vi "_attribute_read_double.vi"(5 "Repeated Capability":string, 7 "Attribute":T1={"Identifier"="", "Descriptive Name"="", "Data Type"=enum."Integer 32", "Command"="", "Access"=enum."Read/Write", "Range Table"="", "Read Callback"="", "Write Callback"="", "Supported Models"="", "Instrument Options"="", "Index"=0, "OPC Wait"=FALSE, "No Status Check"=FALSE, "Cache Only"=FALSE}, 8 "error in":errorcluster caption="error in (no error)", 10 "Query Parameter":string, 11 "VISA resource name":refnum<visa-resource-name>) -> (0 "error out":errorcluster, 2 "Double out":dbl, 3 "VISA resource name out":refnum<visa-resource-name>)   [LabVIEW 2022 SP3, in "hmp4000_rsidr_core.lvlib"]
uses:
  hmp4000_rsidr_core.lvlib
  type_Attribute.ctl
  type_Attribute_Data_Type.ctl
  type_ReadWriteAccess.ctl
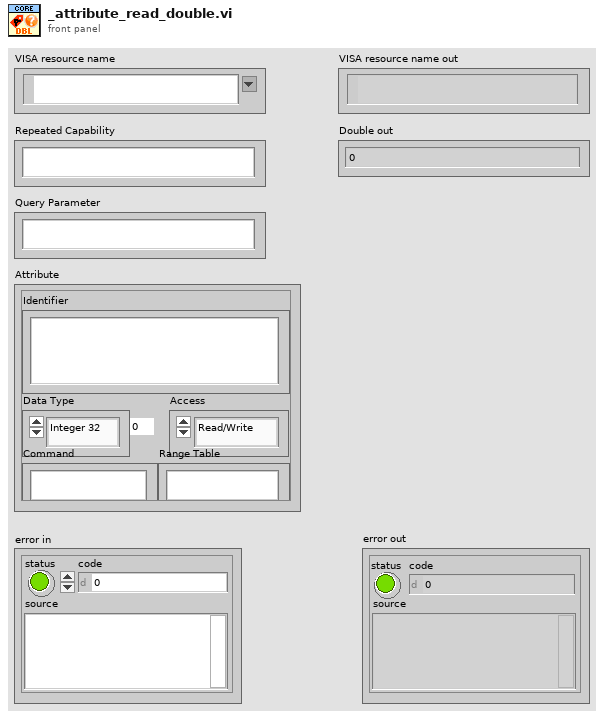
[diagram p1: front panel]
types:
  T1 = typedef "hmp4000_rsidr_core.lvlib/type_Attribute.ctl" = cluster{"Identifier":string, "Descriptive Name":string, "Data Type":T2, "Command":string, "Access":T3, "Range Table":string, "Read Callback":string, "Write Callback":string, "Supported Models":string, "Instrument Options":string, "Index":i32, "OPC Wait":bool, "No Status Check":bool, "Cache Only":bool}
  T2 = typedef "hmp4000_rsidr_core.lvlib/type_Attribute_Data_Type.ctl" = enum16{"Integer 32", "Double", "String", "Boolean", "None", "Integer 64", "RawString"}
  T3 = typedef "hmp4000_rsidr_core.lvlib/type_ReadWriteAccess.ctl" = enum16{"Read Only", "Write Only", "Read/Write"}
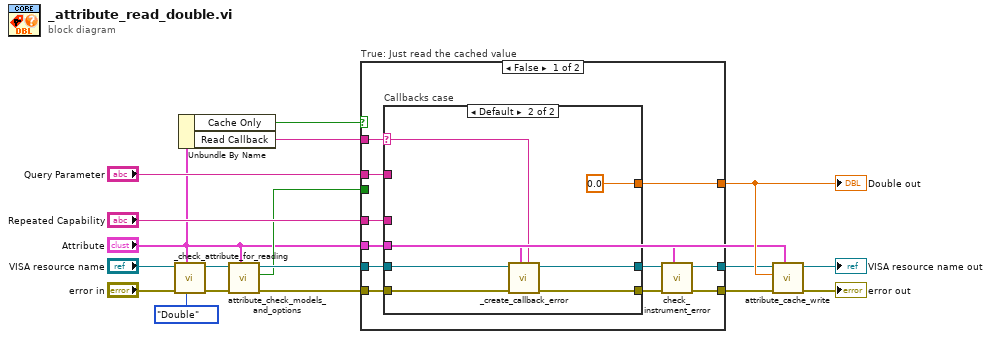
[diagram p0: block diagram]
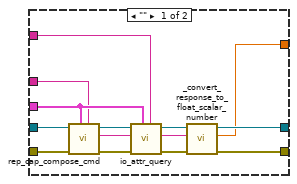
[diagram p2: hidden frame]
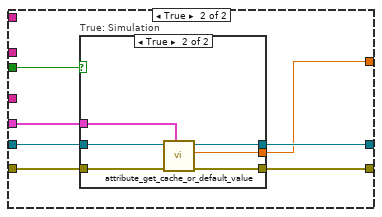
[diagram p3: hidden frame]
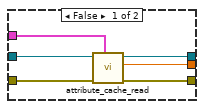
[diagram p4: hidden frame]
diagram:
  n1 = call "_check_attribute_for_reading.vi"("Expected Data Type"=type_Attribute_Data_Type."Double" ("Data Type"), "Attribute"="Attribute", "error in"="error in", "VISA resource name"="VISA resource name") -> ("error out"=w11:errorcluster, "VISA resource name out"=w10:refnum<visa-resource-name>)  [unwired: 6 in]
  n2 = Unbundle By Name("Attribute") -> ("Cache Only"=w1:bool, "Read Callback"=w12:string)
  n3 = call "attribute_check_models_and_options.vi"("Attribute"="Attribute", "error in"=w11, "VISA resource name"=w10) -> ("error out"=w9:errorcluster, "Simulation Mode"=w7:bool, "VISA resource name out"=w8:refnum<visa-resource-name>)  [unwired: 6 in]
  n4 = case "True: Just read the cached value" shown="False" w1 {
    tunnel: "Repeated Capability" -> [w29 _]
    tunnel: [w22 w54] -> w5
    tunnel: [w21 w55] -> w4
    tunnel: [w28 w53] -> w16
    tunnel: w12 -> [w27 _]
    tunnel: w8 -> [w26 w57]
    tunnel: w9 -> [w25 w56]
    tunnel: "Attribute" -> [w23 w52]
    tunnel: w7 -> [_ w51]
    tunnel: "Query Parameter" -> [w24 _]
    frame False {
      n5 = case "Callbacks case" shown="Default" w27 {
        selector: w27 -> [_ w45]
        tunnel: w26 -> [w43 w49]
        tunnel: w25 -> [w42 w50]
        tunnel: w29 -> [w37 _]
        tunnel: [w33 w47] -> w20
        tunnel: [w34 w48] -> w19
        tunnel: [w31 0.0 ("Attribute Value Double")] -> w28
        tunnel: w23 -> [w38 w46]
        tunnel: w24 -> [w30 _]
        frame "" {
          n6 = call "rep_cap_compose_cmd.vi"("Repeated Capability"=w37, "Attribute"=w38, "error in"=w42, "VISA resource name"=w43) -> ("error out"=w41:errorcluster, "Command out"=w40:string, "VISA resource name out"=w39:refnum<visa-resource-name>)  [unwired: 5 in]
          n7 = call "io_attr_query.vi"("Query Parameter (None)"=w30, "Attribute"=w38, "error in"=w41, "write buffer"=w40, "VISA resource name"=w39) -> ("error out"=w36:errorcluster, "read buffer"=w32:string, "VISA resource name out"=w35:refnum<visa-resource-name>)  [unwired: 4 in]
          n8 = call "_convert_response_to_float_scalar_number.vi"("error in"=w36, "Input string"=w32, "VISA resource name"=w35) -> ("error out"=w34:errorcluster, "Double out"=w31:dbl, "VISA resource name out"=w33:refnum<visa-resource-name>)  [unwired: 6 in]
        }
        frame Default {
          n9 = call "_create_callback_error.vi"("Callback Name"=w45, "Attribute"=w46, "error in"=w50, "VISA resource name"=w49) -> ("error out"=w48:errorcluster, "VISA resource name out"=w47:refnum<visa-resource-name>)  [unwired: 6 in]
        }
      }
      n10 = call "check_instrument_error.vi"("Attribute"=w23, "error in"=w19, "VISA resource name"=w20) -> ("error out"=w22:errorcluster, "VISA resource name out"=w21:refnum<visa-resource-name>)  [unwired: 7 in]
    }
    frame True {
      n11 = case "True: Simulation" shown="True" w51 {
        tunnel: w56 -> [w63 w69]
        tunnel: w57 -> [w62 w68]
        tunnel: w52 -> [w61 w65]
        tunnel: [w60 w67] -> w54
        tunnel: [w59 w66] -> w55
        tunnel: [w58 w64] -> w53
        frame False {
          n12 = call "attribute_cache_read.vi"("Attribute"=w61, "error in"=w63, "VISA resource name"=w62) -> ("error out"=w60:errorcluster, "Double out"=w58:dbl, "VISA resource name out"=w59:refnum<visa-resource-name>)  [unwired: 1 in, 5 out]
        }
        frame True {
          n13 = call "attribute_get_cache_or_default_value.vi"("Attribute"=w65, "error in"=w69, "VISA resource name"=w68) -> ("error out"=w67:errorcluster, "Double out"=w64:dbl, "VISA resource name out"=w66:refnum<visa-resource-name>)  [unwired: 1 in, 5 out]
        }
      }
    }
  }
  "Double out" <- w16
  n14 = call "attribute_cache_write.vi"("Attribute"="Attribute", "error in"=w5, "Value in"=w16, "VISA resource name"=w4) -> ("error out"=→"error out":errorcluster, "VISA resource name out"=→"VISA resource name out":refnum<visa-resource-name>)  [unwired: 6 in]
